vi "setupModel.vi"(8 "error in (no error)":errorcluster, 9 "UserEvents in":refnum<class "UserEvents.lvclass">, 11 "Bootloader in":refnum<class "Bootloader.lvclass">) -> (0 "error out":errorcluster, 1 "UserEvents out":refnum<class "UserEvents.lvclass">, 2 "Model out":refnum<class "Model.lvclass">, 3 "Bootloader out":refnum<class "Bootloader.lvclass">)   [LabVIEW 2015, in "Bootloader.lvclass"]
uses:
  Bootloader.lvclass
  Model/Model.lvclass
  UserEvents/UserEvents.lvclass
  Model/Model.lvclass/Model.ctl
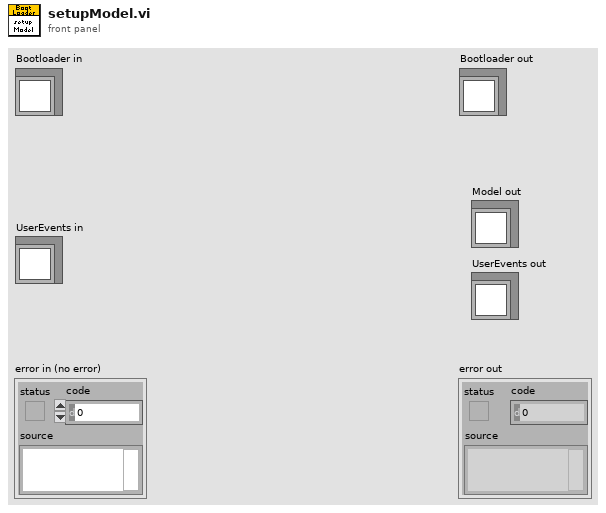
[diagram p1: front panel]
types:
  T1 = typedef "ILCCommon.lvlib/ILCTypedefs.lvlib/Outputs.ctl" = cluster{"Step & Direction":i16, "Blower RPM":u8, "PWM (SSR)":u8, "Ch1":u16, "Ch2":u16, "Ch3":u16, "Ch4":u16}
  T2 = typedef "FAMTTypedefs.lvlib/ForceSensorSettings.ctl" = cluster{"ADC Channel":u8, "Reference Voltage Vref":dbl[unit]}
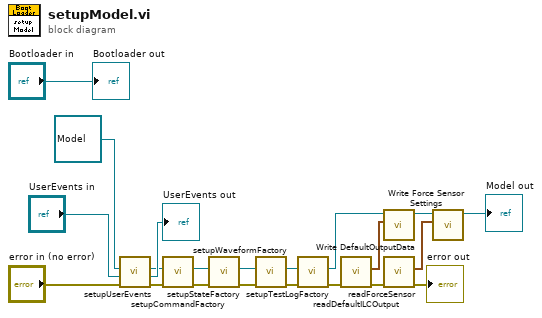
[diagram p0: block diagram]
diagram:
  n1 = call "setupUserEvents.vi"("error in (no error)"="error in (no error)", "UserEvents in"="UserEvents in", "Model in"=refnum<class "Model.lvclass"> refnum) -> ("error out"=w13:errorcluster, "UserEvents out"=→"UserEvents out":refnum<class "UserEvents.lvclass">, "Model out"=w18:refnum<class "Model.lvclass">)  [unwired: 5 in, 1 out]
  n2 = call "setupCommandFactory.vi"("error in (no error)"=w13, "Model in"=w18) -> ("error out"=w12:errorcluster, "Model out"=w17:refnum<class "Model.lvclass">)  [unwired: 7 in, 1 out]
  n3 = call "setupStateFactory.vi"("error in (no error)"=w12, "Model in"=w17) -> ("error out"=w11:errorcluster, "Model out"=w15:refnum<class "Model.lvclass">)  [unwired: 7 in, 1 out]
  n4 = call "setupWaveformFactory.vi"("error in (no error)"=w11, "Model in"=w15) -> ("error out"=w9:errorcluster, "Model out"=w14:refnum<class "Model.lvclass">)  [unwired: 7 in, 1 out]
  n5 = call "setupTestLogFactory.vi"("error in (no error)"=w9, "Model in"=w14) -> ("error out"=w8:errorcluster, "Model out"=w7:refnum<class "Model.lvclass">)  [unwired: 7 in, 1 out]
  n6 = call "readDefaultILCOutput.vi"("error in (no error)"=w8) -> ("error out"=w5:errorcluster, "ILC Outputs"=w6:T1)  [unwired: 8 in, 1 out]
  n7 = call "Write DefaultOutputData.vi"("ILC Outputs"=w6, "Model in"=w7) -> ("Model out"=w4:refnum<class "Model.lvclass">)  [unwired: 9 in]
  n8 = call "readForceSensor.vi"("error in (no error)"=w5) -> ("error out"=→"error out":errorcluster, "Force Sensor Settings"=w2:T2)  [unwired: 8 in, 1 out]
  n9 = call "Write Force Sensor Settings.vi"("Force Sensor Settings"=w2, "Model in"=w4) -> ("Model out"=→"Model out":refnum<class "Model.lvclass">)  [unwired: 9 in]
  "Bootloader out" <- "Bootloader in"
